vi "LocalMode_DSP.vi"(8 "error in (no error)":errorcluster caption="에러 입력(에러 없음)", 11 "VISA resource name":refnum<visa-resource-name>) -> (0 "error out":errorcluster caption="에러 출력", 3 "VISA resource name Out":refnum<visa-resource-name>)   [LabVIEW 2019]
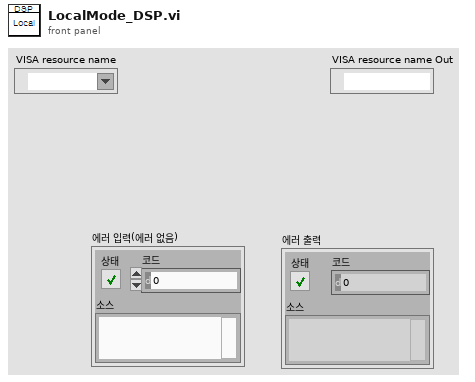
[diagram p1: front panel]
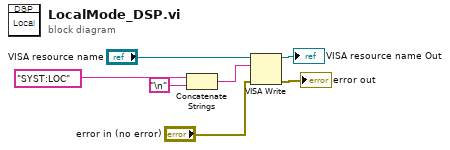
[diagram p0: block diagram]
diagram:
  n1 = Concatenate Strings("SYST:LOC" ("Command"), "\n") -> (w6:string)
  n2 = VISA Write(VISA resource name="VISA resource name", write buffer=w6, error in (no error)="error in (no error)") -> (VISA resource name out=→"VISA resource name Out":refnum<visa-resource-name>, error out=→"error out":errorcluster)  [unwired: 1 out]
